vi "Untitled 5.vi"() -> ()   [LabVIEW 2012]
uses:
  <vilib>/vision/NI_Vision_Development_Module.lvlib
panel:
  out "appended path":path
  out "ROI Descriptor":T1 {"Contours"."Type" items=["No Selection", "Point", "Line", "Rectangle", "Oval", "Polygon", "Freehand Region", "Annulus", "Unused2", "Unused3", "Broken Line", "Freehand Line", "Rotated Rectangle"]}
  out "Read String":string
  in  "Stop":bool
  in  "Delay (s.)":dbl(slide)=0.5079365079365079 scale=0.0..2.0
  out "Image Source":T2(plugin-control)
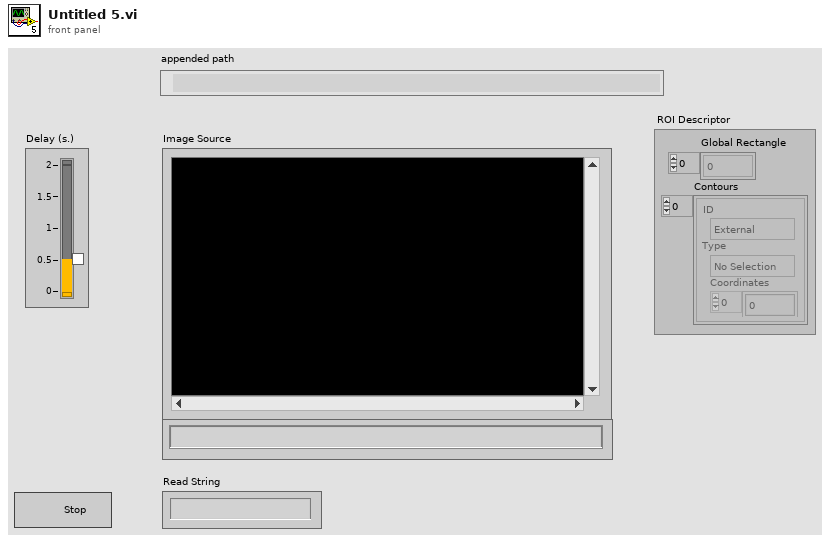
[diagram p1: front panel]
types:
  T1 = typedef "ROI Descriptor" = cluster{"Global Rectangle":i32[], "Contours":cluster{"ID":enum32{"External", "Internal"}, "Type":u32, "Coordinates":i32[]}[]}
  T2 = typedef "IMAQ Image.ctl" = refnum<image>
  T3 = typedef "IMAQ Rectangle" = cluster{"Left":i32, "Top":i32, "Right":i32, "Bottom":i32, "Rotation":dbl}
  T4 = typedef "IMAQ OCR Session.ctl" = refnum<k1>
  T5 = cluster{"Global Rectangle":i32[], "Contours":cluster{"ID":enum32{"External", "Internal"}, "Type":u32, "Coordinates":i32[]}[]}
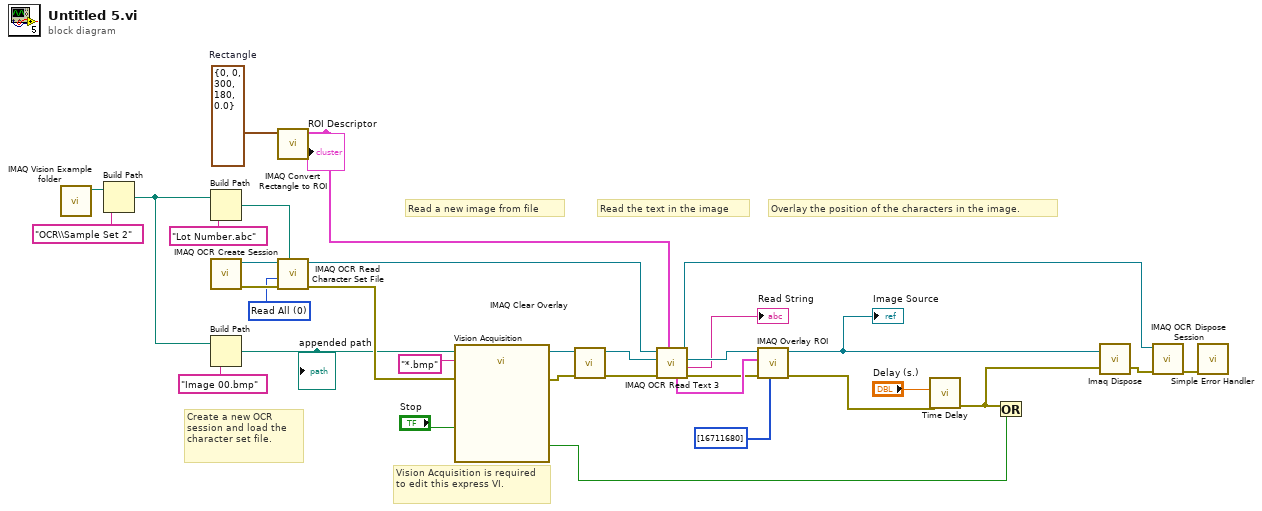
[diagram p0: block diagram]
diagram:
  w26 = T3 {"Left"=0, "Top"=0, "Right"=300, "Bottom"=180, "Rotation"=0.0}  # Rectangle
  w27 = 0 items=["Read All", "Read Character Set Only", "Read Properties Only"] ("Read Options")
  # "Vision Acquisition is required to edit this express VI."
  # "Overlay the position of the characters in the image."
  # "Read the text in the image"
  # "Read a new image from file"
  # "Create a new OCR session and load the character set file."
  n1 = call "IMAQ Vision Example folder.vi"() -> ("Example Image Path"=w31:path)  [unwired: 11 in]
  n2 = Build Path(base path=w31, name or relative path="OCR\\Sample Set 2") -> (appended path=w21:path)
  n3 = Build Path(base path=w21, name or relative path="Lot Number.abc") -> (appended path=w28:path)
  n4 = call "IMAQ OCR Create Session"() -> ("error out"=w29:errorcluster, "IMAQ OCR Session"=w30:T4)  [unwired: 1 in, 9 out]
  n5 = Build Path(base path=w21, name or relative path="Image 00.bmp") -> (appended path=w1:path)
  "appended path" <- w1
  n6 = call "IMAQ Convert Rectangle to ROI"("Rectangle"=w26) -> ("ROI Descriptor"=w25:T1)  [unwired: 8 in, 1 out]
  "ROI Descriptor" <- w25
  n7 = call "IMAQ OCR Read Character Set File"("File Path"=w28, "error in (no error)"=w29, "Read Options"=w27, "IMAQ OCR Session"=w30) -> ("error out"=w20:errorcluster, "IMAQ OCR Session (dup)"=w33:T4)  [unwired: 1 in, 5 out]
  n8 = call "Vision Acquisition"("Image Path"=w1, "Image File Type (All Types)"="*.bmp", "Stop (F)"="Stop", "error in"=w20) -> ("Image Out"=w9:T2, "Stopped"=w5:bool, "error out"=w7:errorcluster)  [unwired: 21 in]
  n9 = call "IMAQ Clear Overlay"("error in (no error)"=w7, "Image"=w9) -> ("error out"=w3:errorcluster, "Image Out"=w8:T2)  [unwired: 1 in, 7 out]
  n10 = call "IMAQ OCR Read Text 3"("ROI Descriptor"=w25, "error in (no error)"=w3, "Image"=w8, "IMAQ OCR Session"=w33) -> ("error out"=w2:errorcluster, "Read String"=→"Read String":string, "Image (dup)"=w13:T2, "IMAQ OCR Session (dup)"=w19:T4, "ROI Bounding Characters"=w15:T5)  [unwired: 1 in, 2 out]
  n11 = call "IMAQ Overlay ROI"("Colors (Green)"=u32[] [16711680], "error in (no error)"=w2, "ROI Descriptor"=w15, "Image"=w13) -> ("error out"=w11:errorcluster, "Image Out"=w24:T2)  [unwired: 2 in, 4 out]
  "Image Source" <- w24
  n12 = call "Time Delay"("error in (no error)"=w11, "Delay Time (s)"="Delay (s.)") -> ("error out"=w23:errorcluster)  [unwired: 9 in]
  n13 = Or(x=w23, y=w5) -> ()  [unwired: 1 out]
  n14 = call "Imaq Dispose"("Image"=w24, "error in (no error)"=w23) -> ("error out"=w17:errorcluster)  [unwired: 1 in, 3 out]
  n15 = call "IMAQ OCR Dispose Session"("error in (no error)"=w17, "IMAQ OCR Session"=w19) -> ("error out"=w18:errorcluster)  [unwired: 9 out]
  n16 = call <vilib>:"Simple Error Handler.vi"("error in (no error)"=w18) -> ()  [unwired: 4 in, 5 out]
